vi "get_prod_name.vi"(8 "error in (no error)":errorcluster, 11 "Resources in":refnum<k20>[](array[refnum])) -> (0 "error out":errorcluster, 1 "Alias":string[](array[string]), 2 "SerialNum":string[](array[string]), 3 "ProdName":string[](array[string]))   [LabVIEW 2015]
uses:
  <resource>/objmgr/nisysapi.rc
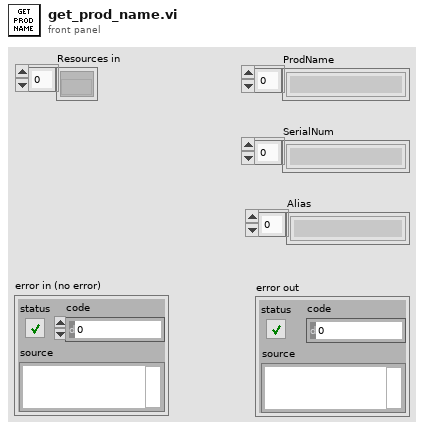
[diagram p1: front panel]
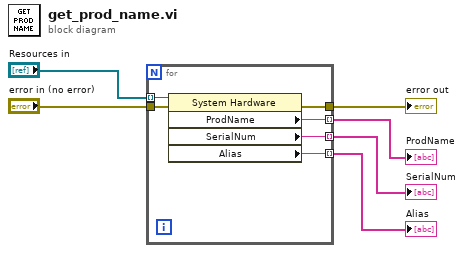
[diagram p0: block diagram]
diagram:
  n1 = for {
    tunnel: "Resources in" -> [w12] mode=indexing
    tunnel: [w11] -> w6 mode=indexing
    tunnel: [w10] -> w5
    tunnel: "error in (no error)" -> [w9]
    tunnel: [w8] -> w2 mode=indexing
    tunnel: [w7] -> w1 mode=indexing
    n2 = property class="System Hardware"(reference=w12, error in=w9) -> (error out=w10:errorcluster, "ProdName"=w11:string, "SerialNum"=w8:string, "Alias"=w7:string)  [unwired: 1 out]
  }
  "ProdName" <- w6
  "error out" <- w5
  "SerialNum" <- w2
  "Alias" <- w1
